vi "motor initialize.vi"(0 "VISA Refnum in":refnum<visa-resource-name>, 1 "DELAY (ms) in":u32, 2 "CONTROLLER":string, 5 "MODE":bool, 7 "MOTOR OFF/ON":bool=TRUE, 9 "CONTINIOUS MODE OFF/ON in":bool, 11 "error in (no error)":errorcluster, 12 "Move Pulse":bool) -> (3 "Dup Controller #":string, 4 "VISA Refnum out":refnum<visa-resource-name>, 6 "DELAY (ms) out":u32, 8 "SELECTED MODE":string, 10 "Response":string, 13 "STATUS":bool, 14 "CONTINIOUS MODE OFF/ON out":bool, 15 "error out":errorcluster)   [LabVIEW 2014]
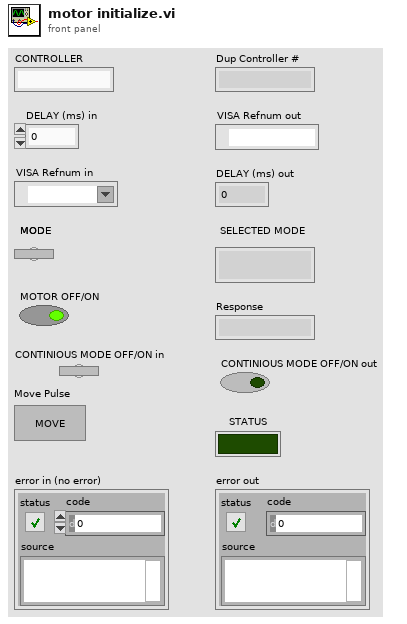
[diagram p1: front panel]
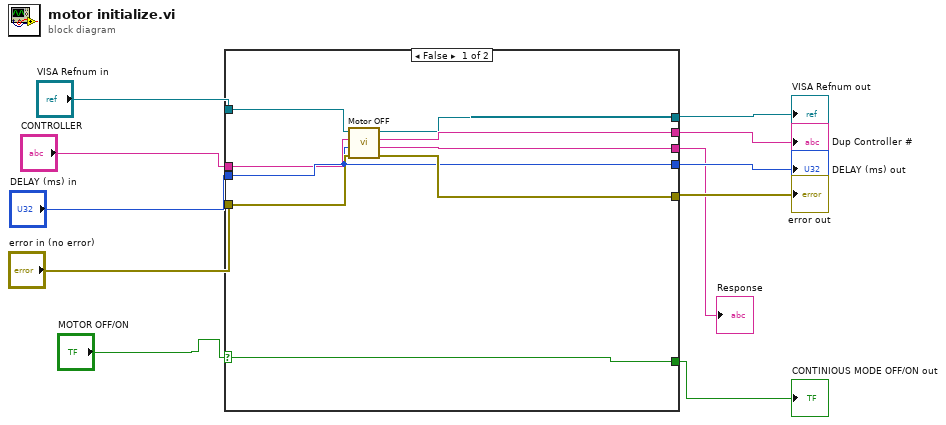
[diagram p0: block diagram]
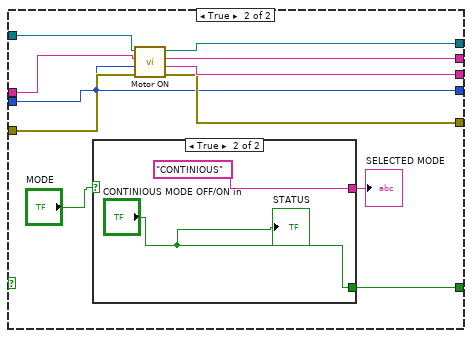
[diagram p2: hidden frame]
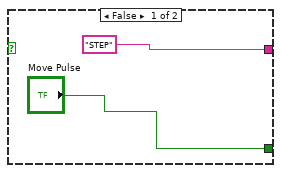
[diagram p3: hidden frame]
diagram:
  n1 = case shown="False" "MOTOR OFF/ON" {
    selector: "MOTOR OFF/ON" -> [w15 _]
    tunnel: "DELAY (ms) in" -> [w14 w23]
    tunnel: "error in (no error)" -> [w20 w31]
    tunnel: [w16 w30] -> w6
    tunnel: [w17 w29] -> w7
    tunnel: [w18 w28] -> w4
    tunnel: [w19 w27] -> w9
    tunnel: [w15 w26] -> w5
    tunnel: [w14 w23] -> w8
    tunnel: "VISA Refnum in" -> [w13 w25]
    tunnel: "CONTROLLER" -> [w12 w24]
    frame False {
      n2 = call <userlib>:"Motor OFF.vi"("error in (no error)"=w20, "Delay (ms)"=w14, "Controller #"=w12, "VISA Handle"=w13) -> ("error out"=w19:errorcluster, "Response"=w18:string, "Dup Controller #"=w17:string, "Dup VISA Handle"=w16:refnum<visa-resource-name>)  [unwired: 2 out]
    }
    frame True {
      n3 = case shown="True" "MODE" {
        tunnel: ["STEP" "CONTINIOUS"] -> w21
        tunnel: ["Move Pulse" "CONTINIOUS MODE OFF/ON in"] -> w26
        frame False {
        }
        frame True {
          "STATUS" <- "CONTINIOUS MODE OFF/ON in"
        }
      }
      "SELECTED MODE" <- w21
      n4 = call <userlib>:"Motor ON.vi"("error in (no error)"=w31, "Delay (ms)"=w23, "Controller #"=w24, "VISA Handle"=w25) -> ("error out"=w27:errorcluster, "Response"=w28:string, "Dup Controller #"=w29:string, "Dup VISA Handle"=w30:refnum<visa-resource-name>)  [unwired: 2 out]
    }
  }
  "error out" <- w9
  "DELAY (ms) out" <- w8
  "Dup Controller #" <- w7
  "VISA Refnum out" <- w6
  "CONTINIOUS MODE OFF/ON out" <- w5
  "Response" <- w4
